vi "Command Type.vi"(11 "Start Log Command Config in":refnum<class "Start Log Command Config.lvclass">) -> (2 "Command Type":T1)   [LabVIEW 2020, in "VolatusSeqConfig.lvlib" / "Start Log Command Config.lvclass"]
uses:
  Start Log Command Config.lvclass
  Start Log Command Config.lvclass/Start Log Command Config.ctl
  Command Type.ctl
  VolatusSeqConfig.lvlib
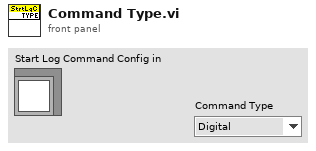
[diagram p1: front panel]
types:
  T1 = typedef "VolatusSeqConfig.lvlib/Command Type.ctl" = enum16{"Digital", "Numeric", "Transition", "Stop", "StartLog", "StopLog"}
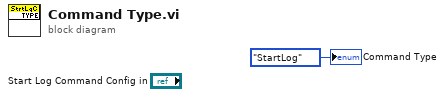
[diagram p0: block diagram]
diagram:
  "Command Type" <- Command_Type."StartLog" ("Command Type")
